vi "set_params.vi"(8 "error in (no error)":errorcluster caption="entrée d'erreur (pas d'erreur)", 11 "Model en entrée":refnum<class "Model.lvclass">) -> (0 "error out":errorcluster caption="sortie d'erreur", 3 "Model en sortie":refnum<class "Model.lvclass">)   [LabVIEW 2020, in "Model.lvclass"]
doc: "Set the parameters of the model."
uses:
  Model.lvclass
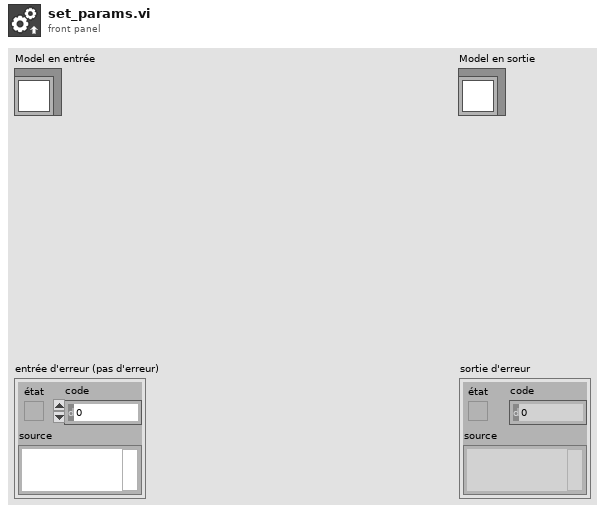
[diagram p1: front panel]
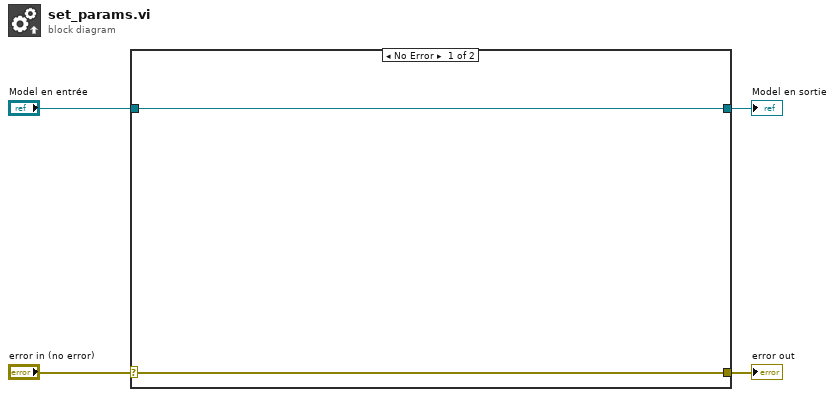
[diagram p0: block diagram]
diagram:
  n1 = case shown="No Error" "error in (no error)" {
    selector: "error in (no error)" -> [w5 w8]
    tunnel: [w5 w8] -> w3
    tunnel: [w6 w7] -> w1
    tunnel: "Model en entrée" -> [w6 w7]
    frame No Error {
    }
    frame Error {
    }
  }
  "error out" <- w3
  "Model en sortie" <- w1
